vi "physical_channels.vi"() -> ()   [LabVIEW 2019]
uses:
  <vilib>/DAQmx/read.llb/DAQmx Read (Analog 2D DBL NChan NSamp).vi
  <vilib>/DAQmx/create/channels.llb/DAQmx Create Channel (AI-Voltage-Basic).vi
  <vilib>/DAQmx/configure/timing.llb/DAQmx Timing (Sample Clock).vi
  <vilib>/DAQmx/miscellaneous.llb/DAQmx Fill In Error Info.vi
panel:
  out "size(s)":i32[](array[numeric])
  out "Waveform Graph":dbl[][](graph)
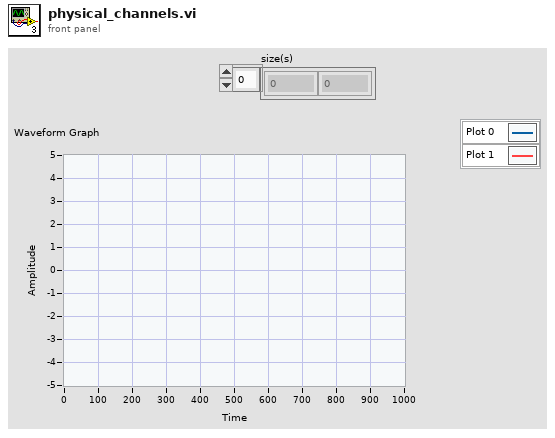
[diagram p1: front panel]
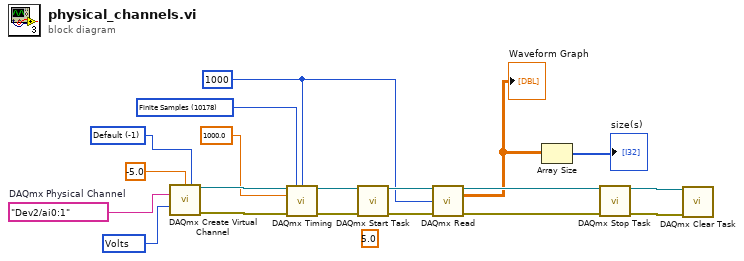
[diagram p0: block diagram]
diagram:
  w3 = 1000 ("samples per channel")
  w4 = 10178 items=["Finite Samples"=10178, "Continuous Samples"=10123, "Hardware Timed Single Point"=12522] ("sample mode")
  w6 = tag "Dev2/ai0:1"  # DAQmx Physical Channel
  w7 = -1 items=["Default"=-1, "RSE"=10083, "NRSE"=10078, "Differential"=10106, "Pseudodifferential"=12529] ("input terminal configuration")
  (unwired) 5.0 ("maximum value")
  w9 = 10348 items=["Volts"=10348, "From Custom Scale"=10065] ("units")
  n1 = call-poly <vilib>:"DAQmx Create Virtual Channel.vi"("minimum value"=-5.0, "input terminal configuration"=w7, "physical channels"=w6, "units"=w9) -> ("task out"=w19:refnum<k21>, "error out"=w18:errorcluster)  [unwired: 10 in]
  n2 = call-poly <vilib>:"DAQmx Timing.vi"("task/channels in"=w19, "sample mode"=w4, "samples per channel"=w3, "rate"=1000.0, "error in"=w18) -> ("task out"=w17:refnum<k21>, "error out"=w16:errorcluster)  [unwired: 9 in]
  n3 = call <vilib>:"DAQmx Start Task.vi"("task/channels in"=w17, "error in"=w16) -> ("task out"=w15:refnum<k21>, "error out"=w14:errorcluster)  [unwired: 12 in]
  n4 = call-poly <vilib>:"DAQmx Read.vi"("task/channels in"=w15, "number of samples per channel"=w3, "error in"=w14) -> ("task out"=w13:refnum<k21>, "data"=w2:dbl[][], "error out"=w12:errorcluster)  [unwired: 10 in]
  "Waveform Graph" <- w2
  n5 = Array Size(array=w2) -> (size(s)=→"size(s)":i32[])
  n6 = call <vilib>:"DAQmx Stop Task.vi"("task/channels in"=w13, "error in"=w12) -> ("task out"=w11:refnum<k21>, "error out"=w10:errorcluster)  [unwired: 12 in]
  n7 = call <vilib>:"DAQmx Clear Task.vi"("task in"=w11, "error in"=w10) -> ()  [unwired: 13 in, 1 out]
